vi "CameraCapture.vi"() -> (3 "Image  out":T1 {"Dialogs" format="%.0b"})   [LabVIEW 2019]
uses:
  <userlib>/ImageProcessing/QTLIB_2595_LV86/QT_Image.ctl
  <userlib>/ImageProcessing/InitCamera_NTSC.vi
panel:
  in  "stop":bool
  out "image":picture
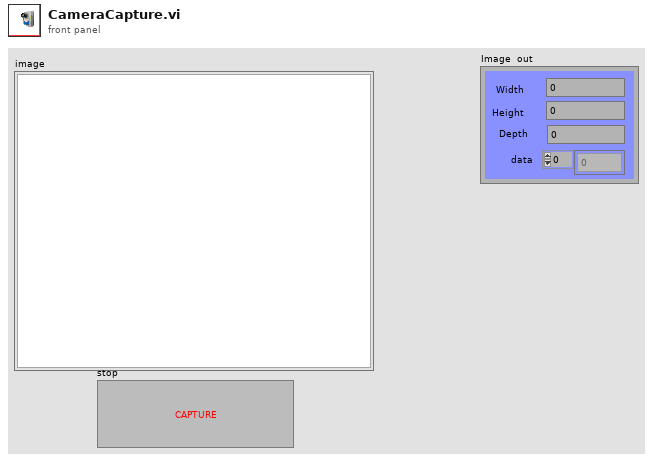
[diagram p1: front panel]
types:
  T1 = typedef "QT_Image.ctl" = cluster{"Width":i32, "Height":i32, "Depth":i32, "data":u8[], "Compressed data":u8[], "Color table":u32[], "Duration":i32, "Options":i32, "Timestamp":i32, "ID":i32, "Reserved":i32, "Dialogs":u32}
  T2 = typedef "QT_Ref.ctl" = refnum<k1>
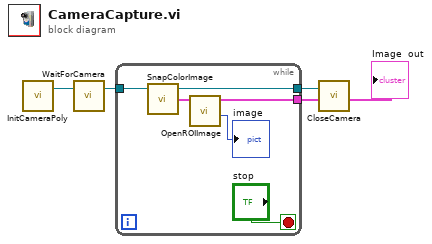
[diagram p0: block diagram]
diagram:
  n1 = call-poly <userlib>:"InitCameraPoly.vi"() -> ("QT Ref Out"=w4:T2)  [unwired: 2 in, 1 out]
  n2 = call <userlib>:"WaitForCamera.vi"("QT Ref In"=w4) -> ("QT Ref Out"=w3:T2)  [unwired: 1 in, 1 out]
  n3 = while {
    tunnel: w3 -> [w10]
    tunnel: [w9] -> w2
    tunnel: [w7] -> w1
    stop <- "stop" stop-if-true
    n4 = call <userlib>:"SnapColorImage.vi"("QT Ref In"=w10) -> ("Image Out"=w8:T1, "QT Ref Out"=w9:T2)  [unwired: 2 in, 1 out]
    n5 = call <userlib>:"OpenROIImage.vi"("Image  in"=w8) -> ("image"=→"image":picture, "Image  out"=w7:T1)  [unwired: 9 in]
  }
  "Image  out" <- w1
  n6 = call <userlib>:"CloseCamera.vi"("QT Ref In"=w2) -> ()  [unwired: 2 in, 1 out]
